vi "Lift Control (SubVI).vi"(10 "Buttons":bool[](array[boolean]), 11 "Lift PID gains":T1={"proportional gain (Kc)"=0.8, "integral time (Ti, min)"=0.01, "derivative time (Td, min)"=0.0} {"derivative time (Td, min)" format="%.3f"; "integral time (Ti, min)" format="%.3f"; "proportional gain (Kc)" format="%.3f"}) -> ()   [LabVIEW 2014]
uses:
  <vilib>/Rock Robotics/WPI/Solenoid/WPI_SolenoidValue.ctl
  <vilib>/Rock Robotics/WPI/Solenoid/WPI_SolenoidSetEnum.vi
  <vilib>/addons/control/pid/pid.llb/PID (DBL).vi
  <vilib>/addons/control/pid/NI_PID_pid.lvlib
panel:
  in  "Lift Speed":dbl=0.7 format="%#_13g"
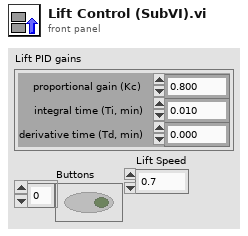
[diagram p1: front panel]
types:
  T1 = cluster{"proportional gain (Kc)":dbl, "integral time (Ti, min)":dbl, "derivative time (Td, min)":dbl}
  T2 = typedef "WPI_SolenoidValue.ctl" = enum16{"Off", "On", "Forward", "Reverse"}
  T3 = typedef "WPI_SwitchDevRef.ctl" = cluster{"DevStatus":errorcluster, "DIO Channel":T4, "Controller":T5, "CntIndex":T6, "Normally Closed":bool}
  T4 = typedef "FPGA_DIOChannel.ctl" = enum8{"DIO 0", "DIO 1", "DIO 2", "DIO 3", "DIO 4", "DIO 5", "DIO 6", "DIO 7", "DIO 8", "DIO 9", "DIO MXP 0", "DIO MXP 1", "DIO MXP 2", "DIO MXP 3", "DIO MXP 4", "DIO MXP 5", "DIO MXP 6", "DIO MXP 7", "DIO MXP 8", "DIO MXP 9", "DIO MXP 10", "DIO MXP 11", "DIO MXP 12", "DIO MXP 13", "DIO MXP 14", "DIO MXP 15", "Invalid"}
  T5 = typedef "FPGA_TypedefDigitalModule.ctl" = enum16{"Controller 1"}
  T6 = typedef "FPGA_CounterCtrSystemIndex.ctl" = enum8{"Ctr 0", "Ctr 1", "Ctr 2", "Ctr 3", "Ctr 4", "Ctr 5", "Ctr 6", "Ctr 7", "Invalid"}
  T7 = typedef "WPI_SolenoidDevRef.ctl" = cluster{"DevStatus":errorcluster, "Pneumatics Control Module":u8, "Forward Solenoid Channel":T8, "Reverse Solenoid Channel":T8}
  T8 = typedef "WPI_SolenoidChannel.ctl" = enum8{"Solenoid 0", "Solenoid 1", "Solenoid 2", "Solenoid 3", "Solenoid 4", "Solenoid 5", "Solenoid 6", "Solenoid 7", "Invalid"}
  T9 = typedef "WPI_MotorControlDeviceRef.ctl" = cluster{"DeviceStatus":errorcluster, "Type":T10, "PWM":cluster{"Controller":T5, "PWM Channel":T11, "DeadBand":T12}, "CAN":cluster{"Device Number":u8, "Control Mode":T13, "Semaphore":T14, "Max Vout":dbl, "TalonSRX Control Mode":T15}, "Invert":bool, "TransformRef":T16, "InvTransformRef":T16}
  T10 = typedef "WPI_MotorControlType.ctl" = enum16{"PWM", "CAN", "CANTalonSRX"}
  T11 = typedef "FPGA_DIOPWMChannel.ctl" = enum8{"PWM 0", "PWM 1", "PWM 2", "PWM 3", "PWM 4", "PWM 5", "PWM 6", "PWM 7", "PWM 8", "PWM 9", "PWM MXP 0", "PWM MXP 1", "PWM MXP 2", "PWM MXP 3", "PWM MXP 4", "PWM MXP 5", "PWM MXP 6", "PWM MXP 7", "PWM MXP 8", "PWM MXP 9", "Invalid"}
  T12 = typedef "WPI_PWMDeadband.ctl" = cluster{"Name":string, "maxPositivePwm":i32, "minPositivePwm":i32, "centerPwm":i32, "maxNegativePwm":i32, "minNegativePwm":i32, "angularRange":u16}
  T13 = typedef "WPI_CANJaguar_ControlMode.ctl" = enum8{"Percent VBus", "Current", "Speed", "Position", "Voltage"}
  T14 = typedef "Semaphore RefNum" = refnum<k1>
  T15 = typedef "WPI_CANTalonSRX_APIControlMode.ctl" = enum8{"Percent VBus", "Speed", "Position", "Slave", "Unchanged / Invalid"}
  T16 = typedef "WPI_PWMTransform_ConPane.ctl" = refnum<vi>
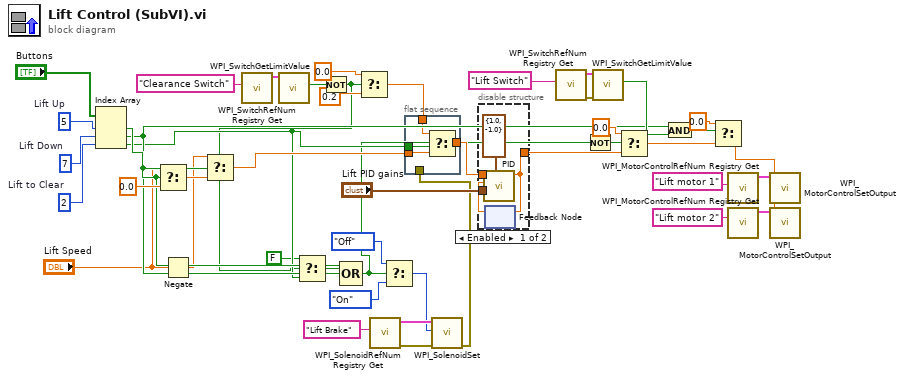
[diagram p0: block diagram]
diagram:
  w46 = 2  # Lift to Clear
  w45 = 7  # Lift Down
  w44 = 5  # Lift Up
  n1 = Index Array(array="Buttons", index #1=w44, index #2=w45, index #3=w46) -> (element #1=w18:bool, element #2=w14:bool, element #3=w10:bool)
  n2 = Select(t="Lift Speed", s=w18, f=0.0) -> (s? t:f=w29:dbl)
  n3 = Negate(x="Lift Speed") -> (-x=w2:dbl)
  n4 = Select(t=w2, s=w14, f=w29) -> (s? t:f=w33:dbl)
  n5 = call <vilib>:"WPI_SwitchRefNum Registry Get.vi"("refnum name"="Clearance Switch") -> ("SwitchDevRef"=w12:T3)  [unwired: 9 in, 1 out]
  n6 = call <vilib>:"WPI_SwitchGetLimitValue.vi"("SwitchDevRef"=w12) -> ("Switch Pressed"=w11:bool)  [unwired: 8 in, 2 out]
  n7 = Not(x=w11) -> (.not. x?=w8:bool)
  n8 = Select(t=FALSE, s=w8, f=w10) -> (s? t:f=w7:bool)
  n9 = Compound Arithmetic op=OR(w18, w14, w7) -> (w5:bool)
  n10 = Select(t=0.0 ("f"), s=w8, f=0.2 ("t")) -> (s? t:f=w36:dbl)
  n11 = call <vilib>:"WPI_SolenoidRefNum Registry Get.vi"("refnum name"="Lift Brake") -> ("error out"=w23:errorcluster, "SolenoidDevRef"=w22:T7)  [unwired: 9 in]
  n12 = Select(t=WPI_SolenoidValue."Off" ("Value"), s=w5, f=WPI_SolenoidValue."On" ("Value")) -> (s? t:f=w19:T2)
  n13 = flat-sequence {
    tunnel: w36 -> [w50]
    tunnel: [w49] -> w34
    tunnel: w33 -> [w48]
    tunnel: w10 -> [w47]
    tunnel: w1 -> [_]
    frame #0 {
      n14 = Select(t=w50, s=w47, f=w48) -> (s? t:f=w49:dbl)
    }
  }
  n15 = call-poly <vilib>:"WPI_SolenoidSet.vi"("error in (no error)"=w23, "Value"=w19, "SolenoidDevRef"=w22) -> ("error out"=w1:errorcluster)  [unwired: 7 in, 1 out]
  n16 = disable-structure shown="Enabled" {
    disable-tunnel: w34 -> [w55 w56]
    disable-tunnel: "Lift PID gains" -> [w53 _]
    disable-tunnel: [w51 w56] -> w17
    frame Enabled {
      n17 = feedback #1() -> (w54:dbl)  [unwired: 1 in]
      n18 = call-poly <vilib>:"PID.vi"("output range"=cluster{"output high":dbl, "output low":dbl} {"output high"=1.0, "output low"=-1.0}, "PID gains"=w53, "process variable"=w54, "setpoint"=w55) -> ("output"=w51:dbl)  [unwired: 6 in, 1 out]
      n19 = feedback-in #1(w51) -> ()
    }
    frame Disabled {
    }
  }
  n20 = call <vilib>:"WPI_SwitchRefNum Registry Get.vi"("refnum name"="Lift Switch") -> ("error out"=w38:errorcluster, "SwitchDevRef"=w39:T3)  [unwired: 9 in]
  n21 = Not(x=w5) -> (.not. x?=w6:bool)
  n22 = call <vilib>:"WPI_SwitchGetLimitValue.vi"("error in (no error)"=w38, "SwitchDevRef"=w39) -> ("Switch Pressed"=w15:bool)  [unwired: 7 in, 2 out]
  n23 = Select(t=0.0, s=w6, f=w17) -> (s? t:f=w41:dbl)
  n24 = And(x=w14, y=w15) -> (x .and. y?=w16:bool)
  n25 = Select(t=0.0, s=w16, f=w41) -> (s? t:f=w42:dbl)
  n26 = call <vilib>:"WPI_MotorControlRefNum Registry Get.vi"("refnum name"="Lift motor 1") -> ("MotorControlDevRef"=w30:T9)  [unwired: 9 in, 1 out]
  n27 = call <vilib>:"WPI_MotorControlRefNum Registry Get.vi"("refnum name"="Lift motor 2") -> ("MotorControlDevRef"=w28:T9)  [unwired: 9 in, 1 out]
  n28 = call <vilib>:"WPI_MotorControlSetOutput.vi"("Output"=w42, "MotorControlDevRef"=w30) -> ()  [unwired: 7 in, 3 out]
  n29 = call <vilib>:"WPI_MotorControlSetOutput.vi"("Output"=w42, "MotorControlDevRef"=w28) -> ()  [unwired: 7 in, 3 out]
